vi "Load DBC.vi"(8 "error in":errorcluster, 10 "Source":string, 11 "Copy of PCAN in":refnum<class "PCAN.lvclass">) -> (0 "error out":errorcluster, 3 "Copy of PCAN out":refnum<class "PCAN.lvclass">)   [LabVIEW 2024, in "PCAN.lvlib" / "PCAN.lvclass"]
uses:
  PCAN.lvclass
  PCAN.lvclass/PCAN.ctl
  <resource>/objmgr/xnet.rc
  <vilib>/xnet/xnet.llb/XNET Create Session (Conversion).vi
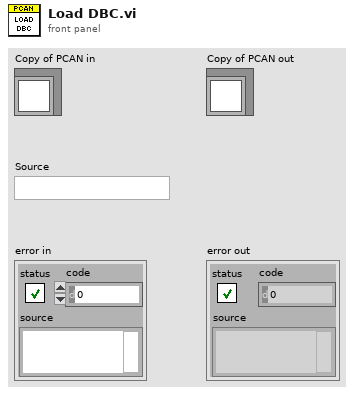
[diagram p1: front panel]
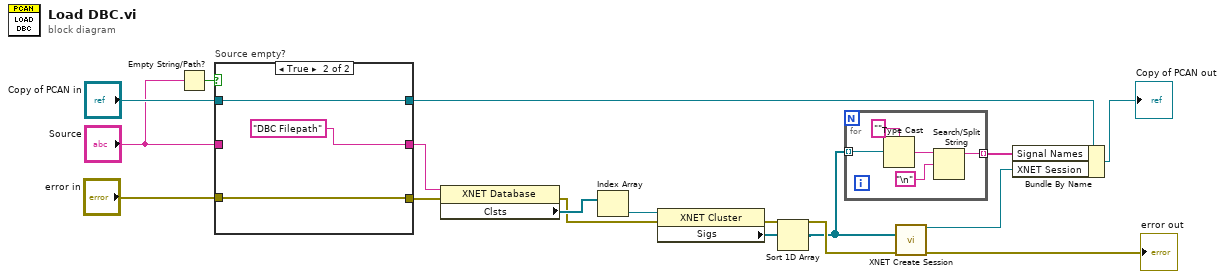
[diagram p0: block diagram]
diagram:
  n1 = Empty String/Path?(string/path="Source") -> (empty?=w2:bool)
  n2 = case "Source empty?" shown="True" w2 {
    tunnel: "Copy of PCAN in" -> [w19 w23]
    tunnel: "error in" -> [w20 w22]
    tunnel: [w18 "DBC Filepath" ("Attribute")] -> w12
    tunnel: [w19 w23] -> w9
    tunnel: [w20 w22] -> w3
    tunnel: "Source" -> [w18 _]
    frame False {
    }
    frame True {
    }
  }
  n3 = property class="XNET Database"(reference=w12, error in=w3) -> (error out=w11:errorcluster, "Clsts"=w13:refnum<k21>[])  [unwired: 1 out]
  n4 = Index Array(array=w13) -> (element=w7:refnum<k21>)  [unwired: 1 in]
  n5 = property class="XNET Cluster"(reference=w7, error in=w11) -> (error out=w6:errorcluster, "Sigs"=w5:refnum<k21>[])  [unwired: 1 out]
  n6 = Sort 1D Array(array=w5) -> (sorted array=w4:refnum<k21>[])
  n7 = for {
    tunnel: w4 -> [w28] mode=indexing
    tunnel: [w25] -> w8 mode=indexing
    n8 = Type Cast(type="", x=w28) -> (*(type *) &x=w26:string)
    n9 = Search/Split String(string=w26, search string/char (-)="\n") -> (substring before match=w25:string)  [unwired: 1 in, 2 out]
  }
  n10 = call-poly <vilib>:"XNET Create Session.vi"("signal list"=w4, "error in (no error)"=w6) -> ("session out"=w10:refnum<k21>, "error out"=→"error out":errorcluster)  [unwired: 12 in]
  n11 = Bundle By Name(cluster=w9, "Signal Names"=w8, "XNET Session"=w10) -> (→"Copy of PCAN out":refnum<class "PCAN.lvclass">)
